vi "scan time(SubVI).vi"(0 "total time":dbl=10.0, 5 "config":T1={"initialize"=enum."SR830", "6221"={"6221 Resource"="GPIB0::24::INSTR", "Delta status"=FALSE, "电流|RMS(A)"=0.0}, "SR830+6221"={"source"=0, "Current(A)"=0.0, "阻抗(Ohm)"=0.0, "SR830 1"=FALSE, "SR830 2"=FALSE, "SR830 3"=FALSE, "SR830 4"=FALSE, "VISA 1"="", "VISA 2"="", "VISA 3"="", "VISA 4"="", "Reserve 1"=0, "Reserve 2"=-1, "Reserve 3"=-1, "Reserve 4"=-1, "Sensitivity 1"=-1, "Sensitivity 2"=0, "Sensitivity 3"=-1, "Sensitivity 4"=-1, "量程入 1"=0, "量程入 2"=0, "量程入 3"=0, "量程入 4"=0}, "2400"={"2400"=FALSE, "VISA"="", "Output Level (0)"=1e-05, "Compliance  Level (0.1)"=10.0, "ch"=[]}, "ch"={"ch"=[], "current"=[], "change?"=[], "holding current\nwhen change ch?"=FALSE}, "Instrument"={"325 Resource "="GPIB0::13::INSTR", "Input (0:A) 325"=0, "Heater Output (1:1) 325"=1, "340 Resource"="GPIB0::14::INSTR", "Input (0:A) 340"=0, "Loop (0: 1)"=0, "Input (0:B) 340"=1, "Loop (1: 1)"=0, "340 Status"=refnum, "Instrument Type"=enum."PPMS-Rotate", "quantum design"=refnum, "semaphore 325"=refnum, "TCP master instance"=refnum, "M24C Resource"="GPIB0::24::INSTR", "4G supply"="GPIB0::24::INSTR", "Temp Status 24C"=refnum, "Temp"=refnum, "9T信号"=refnum, "limit"={"Field limit"=0.0, "Field rate limit"=0.0, "Temp limit"=0.0, "Temp low limit"=0.0, "Temp rate limit "=0.0}, "4g supply status"=refnum, "vi路径"="", "in-plane"="", "out-plane"="", "in-plane signal"=FALSE, "out-plane signal"=FALSE, "in plane 信号"=refnum, "pzt volt"=refnum, "Aborting"=refnum, "数据文件"=refnum, "warning"=refnum, "750 visa"="", "750 rotate"="", "335 Status 2"=refnum, "335 Resource "="GPIB0::24::INSTR", "Input (0:A) 335"=0, "Input (0:B) 335"=1, "Heater Output (1:1) 335"=1, "semaphore 340"=refnum, "semaphore 335"=refnum, "325 Status"=refnum, "semaphore 750"=refnum, "750 field status"=refnum, "camg 振荡状态"=refnum, "列表框"=refnum, "编辑列表框？"=refnum, "camg Rate"=refnum, "行数"=refnum, "TM620"="TCPIP0::192.168.1.5::4266::SOCKET"}, "2614B"={"2614B chA"=FALSE, "2614B chB"=FALSE, "VISA"=""}, "33522b"={"33522b resource name"="", "零电压"=0.0, "最大电压"=148.0, "间隔"=4.0, "最小电压"=-48.0, "loop"=0.0}, "gating type"=enum."2614(daul)", "层数"=0, "行数"=0, "是否处理"=[]} {"Instrument"."Loop (1: 1)" items=["1"=1, "2"=2]; "Instrument"."Loop (0: 1)" items=["1"=1, "2"=2]; "Instrument"."Input (0:B) 340" items=["A", "B", "C", "D"]; "Instrument"."Heater Output (1:1) 335" items=["1"=1, "2"=2]; "Instrument"."Input (0:B) 335" items=["A", "B"]; "Instrument"."Input (0:A) 335" items=["A", "B"]; "Instrument"."Heater Output (1:1) 325" items=["1"=1, "2"=2]; "Instrument"."Input (0:A) 325" items=["A", "B"]; "Instrument"."Input (0:A) 340" items=["1"=1, "2"=2]; "SR830+6221"."Sensitivity 4" items=["Auto Gain"=-1, "2 nV/fA"=0, "5 nV/fA"=1, "10 nV/fA"=2, "20 nV/fA"=3, "50 nV/fA"=4, "100 nV/fA"=5, "200 nV/fA"=6, "500 nV/fA"=7, "1 uV/pA"=8, "2 uV/pA"=9, "5 uV/pA"=10, "10 uV/pA"=11, "20 uV/pA"=12, "50 uV/pA"=13, "100 uV/pA"=14, "200 uV/pA"=15, "500 uV/pA"=16, "1 mV/nA"=17, "2 mV/nA"=18, "5 mV/nA"=19, "10 mV/nA"=20, "20 mV/nA"=21, "50 mV/nA"=22, "100 mV/nA"=23, "200 mV/nA"=24, "500 mV/mA"=25, "1 V/uA"=26]; "SR830+6221"."Sensitivity 3" items=["Auto Gain"=-1, "2 nV/fA"=0, "5 nV/fA"=1, "10 nV/fA"=2, "20 nV/fA"=3, "50 nV/fA"=4, "100 nV/fA"=5, "200 nV/fA"=6, "500 nV/fA"=7, "1 uV/pA"=8, "2 uV/pA"=9, "5 uV/pA"=10, "10 uV/pA"=11, "20 uV/pA"=12, "50 uV/pA"=13, "100 uV/pA"=14, "200 uV/pA"=15, "500 uV/pA"=16, "1 mV/nA"=17, "2 mV/nA"=18, "5 mV/nA"=19, "10 mV/nA"=20, "20 mV/nA"=21, "50 mV/nA"=22, "100 mV/nA"=23, "200 mV/nA"=24, "500 mV/mA"=25, "1 V/uA"=26]; "SR830+6221"."Sensitivity 1" items=["Auto Gain"=-1, "2 nV/fA"=0, "5 nV/fA"=1, "10 nV/fA"=2, "20 nV/fA"=3, "50 nV/fA"=4, "100 nV/fA"=5, "200 nV/fA"=6, "500 nV/fA"=7, "1 uV/pA"=8, "2 uV/pA"=9, "5 uV/pA"=10, "10 uV/pA"=11, "20 uV/pA"=12, "50 uV/pA"=13, "100 uV/pA"=14, "200 uV/pA"=15, "500 uV/pA"=16, "1 mV/nA"=17, "2 mV/nA"=18, "5 mV/nA"=19, "10 mV/nA"=20, "20 mV/nA"=21, "50 mV/nA"=22, "100 mV/nA"=23, "200 mV/nA"=24, "500 mV/mA"=25, "1 V/uA"=26]; "SR830+6221"."Sensitivity 2" items=["Auto Gain"=-1, "2 nV/fA"=0, "5 nV/fA"=1, "10 nV/fA"=2, "20 nV/fA"=3, "50 nV/fA"=4, "100 nV/fA"=5, "200 nV/fA"=6, "500 nV/fA"=7, "1 uV/pA"=8, "2 uV/pA"=9, "5 uV/pA"=10, "10 uV/pA"=11, "20 uV/pA"=12, "50 uV/pA"=13, "100 uV/pA"=14, "200 uV/pA"=15, "500 uV/pA"=16, "1 mV/nA"=17, "2 mV/nA"=18, "5 mV/nA"=19, "10 mV/nA"=20, "20 mV/nA"=21, "50 mV/nA"=22, "100 mV/nA"=23, "200 mV/nA"=24, "500 mV/mA"=25, "1 V/uA"=26]; "SR830+6221"."Reserve 4" items=["Auto Gain"=-1, "2 nV/fA"=0, "5 nV/fA"=1, "10 nV/fA"=2, "20 nV/fA"=3, "50 nV/fA"=4, "100 nV/fA"=5, "200 nV/fA"=6, "500 nV/fA"=7, "1 uV/pA"=8, "2 uV/pA"=9, "5 uV/pA"=10, "10 uV/pA"=11, "20 uV/pA"=12, "50 uV/pA"=13, "100 uV/pA"=14, "200 uV/pA"=15, "500 uV/pA"=16, "1 mV/nA"=17, "2 mV/nA"=18, "5 mV/nA"=19, "10 mV/nA"=20, "20 mV/nA"=21, "50 mV/nA"=22, "100 mV/nA"=23, "200 mV/nA"=24, "500 mV/mA"=25, "1 V/uA"=26]; "SR830+6221"."Reserve 3" items=["Auto Reserve"=-1, "High Reserve"=0, "Normal"=1, "Low Noise"=2]; "SR830+6221"."Reserve 2" items=["Auto Reserve"=-1, "High Reserve"=0, "Normal"=1, "Low Noise"=2]; "SR830+6221"."Reserve 1" items=["Auto Reserve"=-1, "High Reserve"=0, "Normal"=1, "Low Noise"=2]; "SR830+6221"."source" items=["SR830 1", "SR830 2", "SR830 3", "SR830 4"]}, 9 "steps number":i32, 12 "data":refnum<queue>) -> (4 "输出簇":T1={"initialize"=enum."SR830", "6221"={"6221 Resource"="GPIB0::24::INSTR", "Delta status"=FALSE, "电流|RMS(A)"=0.0}, "SR830+6221"={"source"=0, "Current(A)"=0.0, "阻抗(Ohm)"=0.0, "SR830 1"=FALSE, "SR830 2"=FALSE, "SR830 3"=FALSE, "SR830 4"=FALSE, "VISA 1"="", "VISA 2"="", "VISA 3"="", "VISA 4"="", "Reserve 1"=0, "Reserve 2"=-1, "Reserve 3"=-1, "Reserve 4"=-1, "Sensitivity 1"=-1, "Sensitivity 2"=0, "Sensitivity 3"=-1, "Sensitivity 4"=-1, "量程入 1"=0, "量程入 2"=0, "量程入 3"=0, "量程入 4"=0}, "2400"={"2400"=FALSE, "VISA"="", "Output Level (0)"=1e-05, "Compliance  Level (0.1)"=10.0, "ch"=[]}, "ch"={"ch"=[], "current"=[], "change?"=[], "holding current\nwhen change ch?"=FALSE}, "Instrument"={"325 Resource "="GPIB0::13::INSTR", "Input (0:A) 325"=0, "Heater Output (1:1) 325"=1, "340 Resource"="GPIB0::14::INSTR", "Input (0:A) 340"=0, "Loop (0: 1)"=0, "Input (0:B) 340"=1, "Loop (1: 1)"=0, "340 Status"=refnum, "Instrument Type"=enum."PPMS-Rotate", "quantum design"=refnum, "semaphore 325"=refnum, "TCP master instance"=refnum, "M24C Resource"="GPIB0::24::INSTR", "4G supply"="GPIB0::24::INSTR", "Temp Status 24C"=refnum, "Temp"=refnum, "9T信号"=refnum, "limit"={"Field limit"=0.0, "Field rate limit"=0.0, "Temp limit"=0.0, "Temp low limit"=0.0, "Temp rate limit "=0.0}, "4g supply status"=refnum, "vi路径"="", "in-plane"="", "out-plane"="", "in-plane signal"=FALSE, "out-plane signal"=FALSE, "in plane 信号"=refnum, "pzt volt"=refnum, "Aborting"=refnum, "数据文件"=refnum, "warning"=refnum, "750 visa"="", "750 rotate"="", "335 Status 2"=refnum, "335 Resource "="GPIB0::24::INSTR", "Input (0:A) 335"=0, "Input (0:B) 335"=1, "Heater Output (1:1) 335"=1, "semaphore 340"=refnum, "semaphore 335"=refnum, "325 Status"=refnum, "semaphore 750"=refnum, "750 field status"=refnum, "camg 振荡状态"=refnum, "列表框"=refnum, "编辑列表框？"=refnum, "camg Rate"=refnum, "行数"=refnum, "TM620"="TCPIP0::192.168.1.5::4266::SOCKET"}, "2614B"={"2614B chA"=FALSE, "2614B chB"=FALSE, "VISA"=""}, "33522b"={"33522b resource name"="", "零电压"=0.0, "最大电压"=148.0, "间隔"=4.0, "最小电压"=-48.0, "loop"=0.0}, "gating type"=enum."2614(daul)", "层数"=0, "行数"=0, "是否处理"=[]} {"Instrument"."Loop (1: 1)" items=["1"=1, "2"=2]; "Instrument"."Loop (0: 1)" items=["1"=1, "2"=2]; "Instrument"."Input (0:B) 340" items=["A", "B", "C", "D"]; "Instrument"."Heater Output (1:1) 335" items=["1"=1, "2"=2]; "Instrument"."Input (0:B) 335" items=["A", "B"]; "Instrument"."Input (0:A) 335" items=["A", "B"]; "Instrument"."Heater Output (1:1) 325" items=["1"=1, "2"=2]; "Instrument"."Input (0:A) 325" items=["A", "B"]; "Instrument"."Input (0:A) 340" items=["1"=1, "2"=2]; "SR830+6221"."Sensitivity 4" items=["Auto Gain"=-1, "2 nV/fA"=0, "5 nV/fA"=1, "10 nV/fA"=2, "20 nV/fA"=3, "50 nV/fA"=4, "100 nV/fA"=5, "200 nV/fA"=6, "500 nV/fA"=7, "1 uV/pA"=8, "2 uV/pA"=9, "5 uV/pA"=10, "10 uV/pA"=11, "20 uV/pA"=12, "50 uV/pA"=13, "100 uV/pA"=14, "200 uV/pA"=15, "500 uV/pA"=16, "1 mV/nA"=17, "2 mV/nA"=18, "5 mV/nA"=19, "10 mV/nA"=20, "20 mV/nA"=21, "50 mV/nA"=22, "100 mV/nA"=23, "200 mV/nA"=24, "500 mV/mA"=25, "1 V/uA"=26]; "SR830+6221"."Sensitivity 3" items=["Auto Gain"=-1, "2 nV/fA"=0, "5 nV/fA"=1, "10 nV/fA"=2, "20 nV/fA"=3, "50 nV/fA"=4, "100 nV/fA"=5, "200 nV/fA"=6, "500 nV/fA"=7, "1 uV/pA"=8, "2 uV/pA"=9, "5 uV/pA"=10, "10 uV/pA"=11, "20 uV/pA"=12, "50 uV/pA"=13, "100 uV/pA"=14, "200 uV/pA"=15, "500 uV/pA"=16, "1 mV/nA"=17, "2 mV/nA"=18, "5 mV/nA"=19, "10 mV/nA"=20, "20 mV/nA"=21, "50 mV/nA"=22, "100 mV/nA"=23, "200 mV/nA"=24, "500 mV/mA"=25, "1 V/uA"=26]; "SR830+6221"."Sensitivity 1" items=["Auto Gain"=-1, "2 nV/fA"=0, "5 nV/fA"=1, "10 nV/fA"=2, "20 nV/fA"=3, "50 nV/fA"=4, "100 nV/fA"=5, "200 nV/fA"=6, "500 nV/fA"=7, "1 uV/pA"=8, "2 uV/pA"=9, "5 uV/pA"=10, "10 uV/pA"=11, "20 uV/pA"=12, "50 uV/pA"=13, "100 uV/pA"=14, "200 uV/pA"=15, "500 uV/pA"=16, "1 mV/nA"=17, "2 mV/nA"=18, "5 mV/nA"=19, "10 mV/nA"=20, "20 mV/nA"=21, "50 mV/nA"=22, "100 mV/nA"=23, "200 mV/nA"=24, "500 mV/mA"=25, "1 V/uA"=26]; "SR830+6221"."Sensitivity 2" items=["Auto Gain"=-1, "2 nV/fA"=0, "5 nV/fA"=1, "10 nV/fA"=2, "20 nV/fA"=3, "50 nV/fA"=4, "100 nV/fA"=5, "200 nV/fA"=6, "500 nV/fA"=7, "1 uV/pA"=8, "2 uV/pA"=9, "5 uV/pA"=10, "10 uV/pA"=11, "20 uV/pA"=12, "50 uV/pA"=13, "100 uV/pA"=14, "200 uV/pA"=15, "500 uV/pA"=16, "1 mV/nA"=17, "2 mV/nA"=18, "5 mV/nA"=19, "10 mV/nA"=20, "20 mV/nA"=21, "50 mV/nA"=22, "100 mV/nA"=23, "200 mV/nA"=24, "500 mV/mA"=25, "1 V/uA"=26]; "SR830+6221"."Reserve 4" items=["Auto Gain"=-1, "2 nV/fA"=0, "5 nV/fA"=1, "10 nV/fA"=2, "20 nV/fA"=3, "50 nV/fA"=4, "100 nV/fA"=5, "200 nV/fA"=6, "500 nV/fA"=7, "1 uV/pA"=8, "2 uV/pA"=9, "5 uV/pA"=10, "10 uV/pA"=11, "20 uV/pA"=12, "50 uV/pA"=13, "100 uV/pA"=14, "200 uV/pA"=15, "500 uV/pA"=16, "1 mV/nA"=17, "2 mV/nA"=18, "5 mV/nA"=19, "10 mV/nA"=20, "20 mV/nA"=21, "50 mV/nA"=22, "100 mV/nA"=23, "200 mV/nA"=24, "500 mV/mA"=25, "1 V/uA"=26]; "SR830+6221"."Reserve 3" items=["Auto Reserve"=-1, "High Reserve"=0, "Normal"=1, "Low Noise"=2]; "SR830+6221"."Reserve 2" items=["Auto Reserve"=-1, "High Reserve"=0, "Normal"=1, "Low Noise"=2]; "SR830+6221"."Reserve 1" items=["Auto Reserve"=-1, "High Reserve"=0, "Normal"=1, "Low Noise"=2]; "SR830+6221"."source" items=["SR830 1", "SR830 2", "SR830 3", "SR830 4"]}, 6 "错误输出":errorcluster)   [LabVIEW 2019, in "Scan.lvlib"]
uses:
  Scan.lvlib
  ctl/config.ctl
  <vilib>/NI/Modbus Library/API/Master/Modbus Master.lvclass
  ctl/initialize.ctl
  ctl/Instrument.ctl
  ctl/335 state.ctl
  ctl/Instrument Type.ctl
  C:/Users/fuyang/Desktop/postdoctor/labview/labview-measure/lib/QDInstrument.dll
  lib/QDInstrument.dll
  ctl/limit.ctl
  ctl/9T mag field stauts.ctl
  ctl/warning.ctl
  ctl/Gating type.ctl
  User lib.lvlib
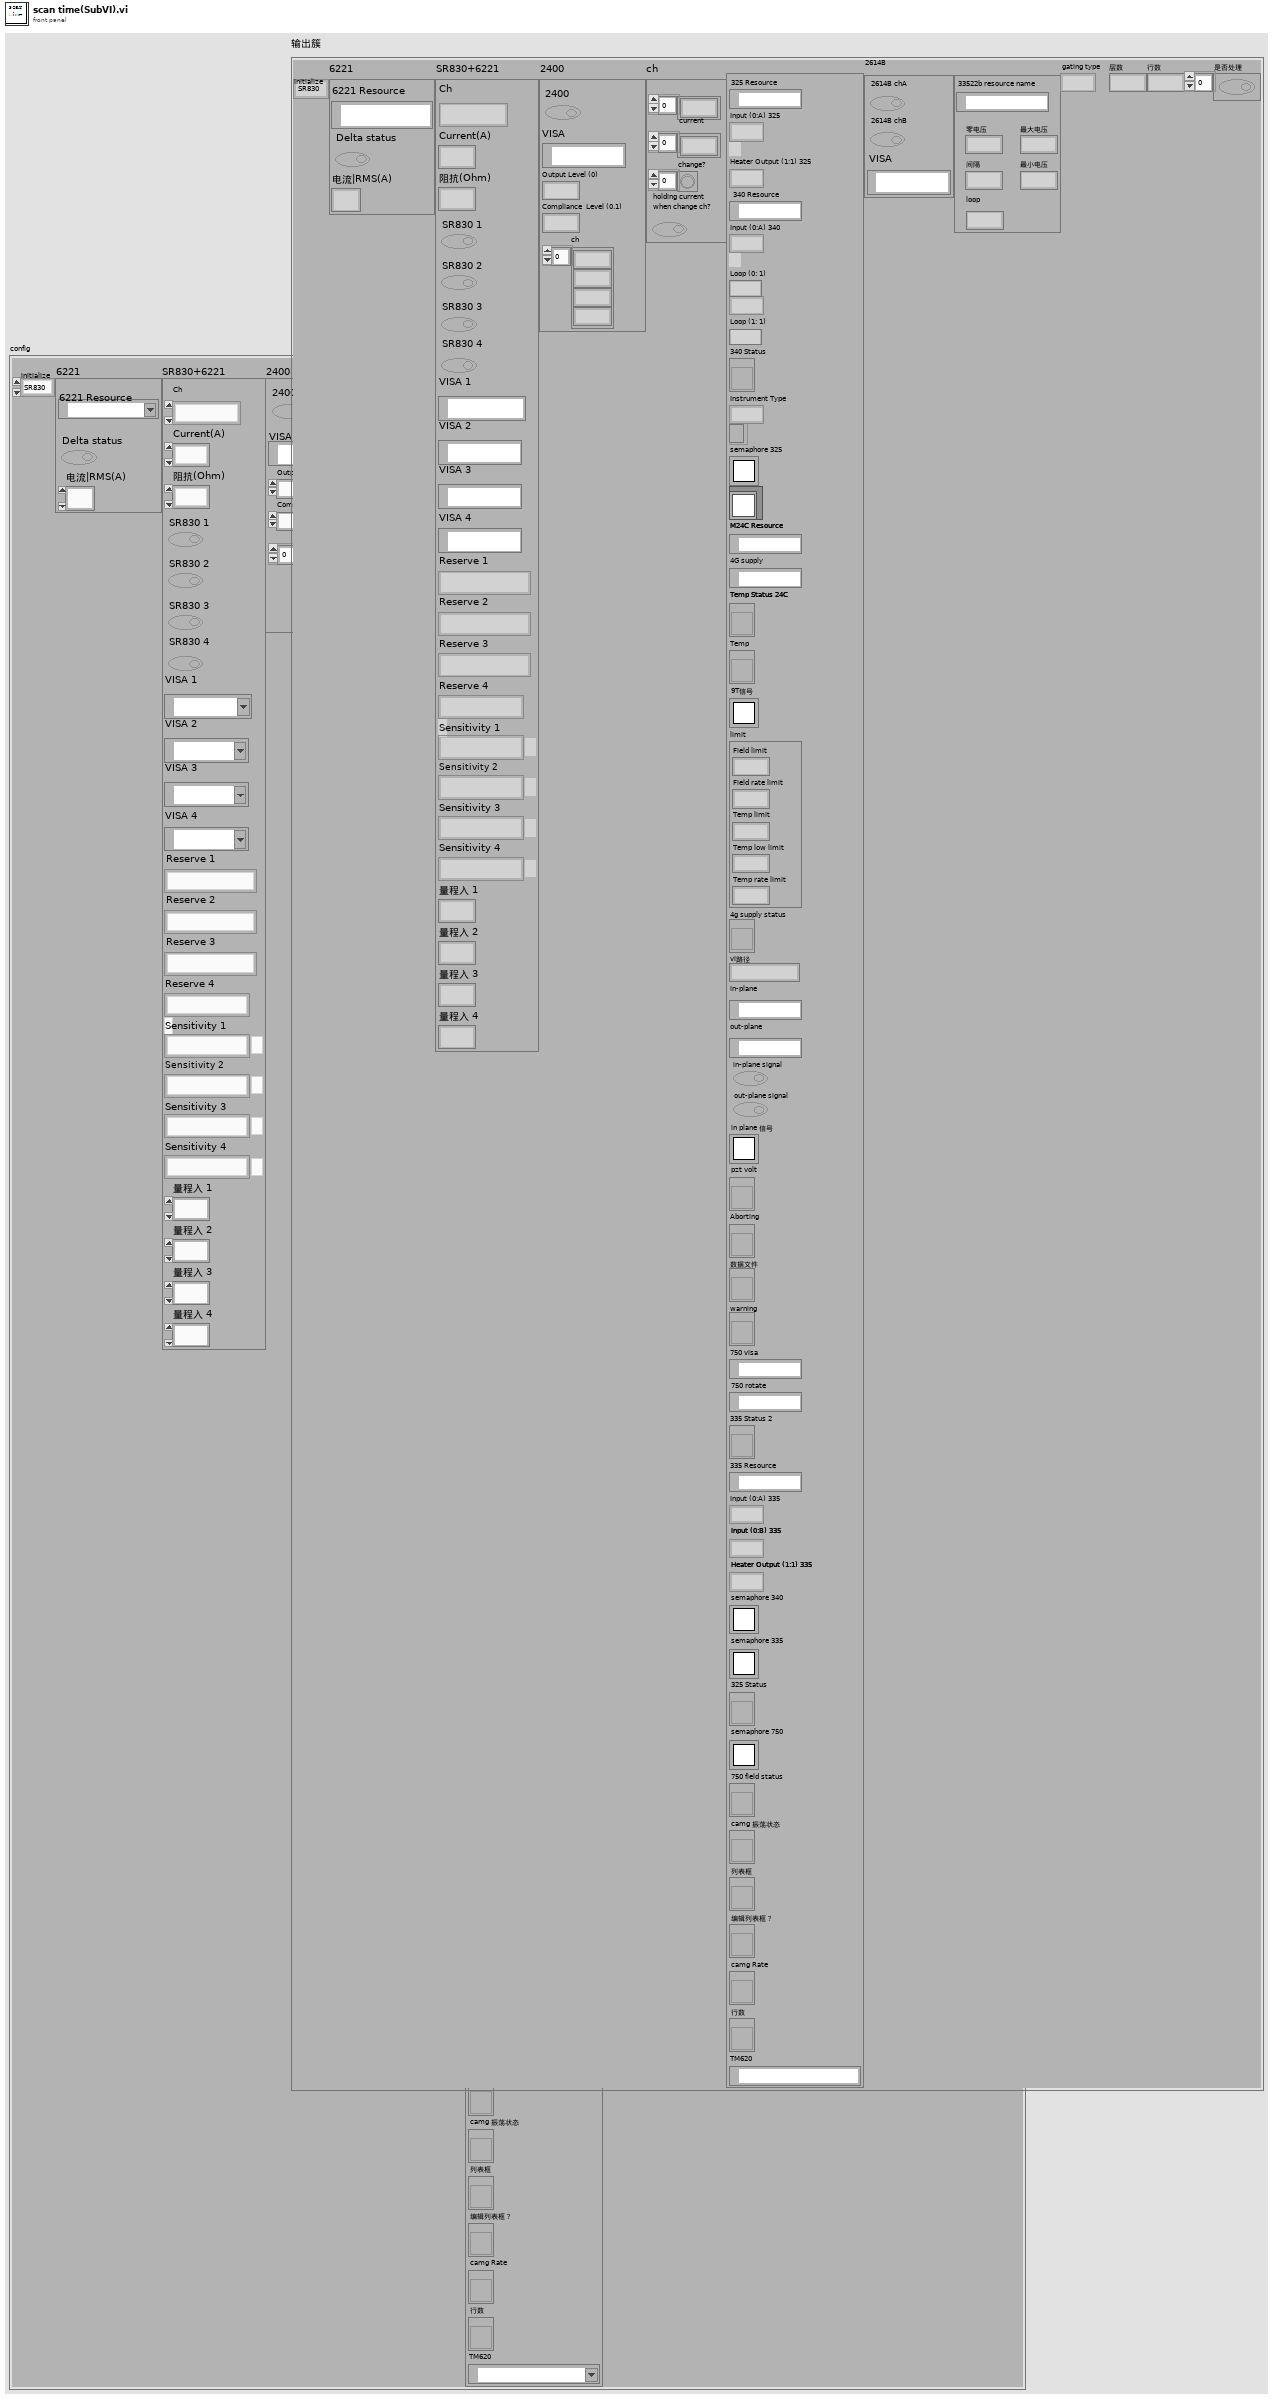
[diagram p1: front panel]
types:
  T1 = typedef "config.ctl" = cluster{"initialize":T2, "6221":cluster{"6221 Resource":refnum<visa-resource-name>, "Delta status":bool, "电流|RMS(A)":dbl}, "SR830+6221":cluster{"source":u16, "Current(A)":dbl, "阻抗(Ohm)":dbl, "SR830 1":bool, "SR830 2":bool, "SR830 3":bool, "SR830 4":bool, "VISA 1":refnum<visa-resource-name>, "VISA 2":refnum<visa-resource-name>, "VISA 3":refnum<visa-resource-name>, "VISA 4":refnum<visa-resource-name>, "Reserve 1":i16, "Reserve 2":i16, "Reserve 3":i16, "Reserve 4":i16, "Sensitivity 1":i16, "Sensitivity 2":i16, "Sensitivity 3":i16, "Sensitivity 4":i16, "量程入 1":i32, "量程入 2":i32, "量程入 3":i32, "量程入 4":i32}, "2400":cluster{"2400":bool, "VISA":refnum<visa-resource-name>, "Output Level (0)":dbl, "Compliance  Level (0.1)":dbl, "ch":i32[]}, "ch":cluster{"ch":i32[], "current":dbl[], "change?":bool[], "holding current\nwhen change ch?":bool}, "Instrument":T3, "2614B":cluster{"2614B chA":bool, "2614B chB":bool, "VISA":refnum<visa-resource-name>}, "33522b":cluster{"33522b resource name":refnum<visa-resource-name>, "零电压":dbl, "最大电压":dbl, "间隔":dbl, "最小电压":dbl, "loop":dbl}, "gating type":T7, "层数":i32, "行数":i32, "是否处理":bool[]}
  T2 = typedef "initialize.ctl" = enum16{"SR830", "keithley6221-SR830", "Delta", "Delta-tunnelling", "keithley6221-2182-DC", "PZT", "4200"}
  T3 = typedef "Instrument.ctl" = cluster{"325 Resource ":refnum<visa-resource-name>, "Input (0:A) 325":u16, "Heater Output (1:1) 325":u16, "340 Resource":refnum<visa-resource-name>, "Input (0:A) 340":u16, "Loop (0: 1)":u16, "Input (0:B) 340":u16, "Loop (1: 1)":u16, "340 Status":refnum<vi>, "Instrument Type":T4, "quantum design":refnum<k24>, "semaphore 325":T5, "TCP master instance":refnum<class "Modbus Master.lvclass">, "M24C Resource":refnum<visa-resource-name>, "4G supply":refnum<visa-resource-name>, "Temp Status 24C":refnum<vi>, "Temp":refnum<vi>, "9T信号":T5, "limit":T6, "4g supply status":refnum<vi>, "vi路径":string, "in-plane":refnum<visa-resource-name>, "out-plane":refnum<visa-resource-name>, "in-plane signal":bool, "out-plane signal":bool, "in plane 信号":T5, "pzt volt":refnum<vi>, "Aborting":refnum<vi>, "数据文件":refnum<vi>, "warning":refnum<vi>, "750 visa":refnum<visa-resource-name>, "750 rotate":refnum<visa-resource-name>, "335 Status 2":refnum<vi>, "335 Resource ":refnum<visa-resource-name>, "Input (0:A) 335":u16, "Input (0:B) 335":u16, "Heater Output (1:1) 335":u16, "semaphore 340":T5, "semaphore 335":T5, "325 Status":refnum<vi>, "semaphore 750":T5, "750 field status":refnum<vi>, "camg 振荡状态":refnum<vi>, "列表框":refnum<vi>, "编辑列表框？":refnum<vi>, "camg Rate":refnum<vi>, "行数":refnum<vi>, "TM620":refnum<visa-resource-name>}
  T4 = typedef "Instrument Type.ctl" = enum16{"PPMS", "VersaLab", "DynaCool", "SVSM", "PPMS-Rotate", "Lakeshore335", "lengtou2", "9T mag old", "9T cmag", "9T cmag DAC", "9T cmag rotate", "test"}
  T5 = typedef "Semaphore RefNum" = refnum<k1>
  T6 = typedef "limit.ctl" = cluster{"Field limit":dbl, "Field rate limit":dbl, "Temp limit":dbl, "Temp low limit":dbl, "Temp rate limit ":dbl}
  T7 = typedef "Gating type.ctl" = enum32{"null", "2614(daul)", "2400", "6517B"}
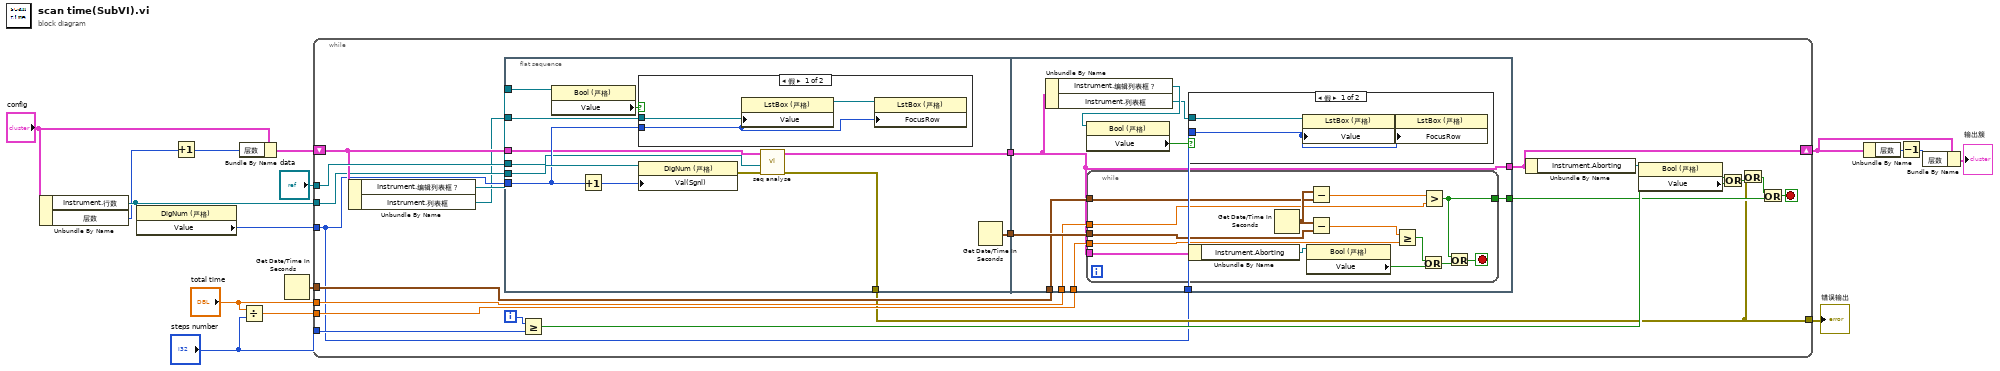
[diagram p0: block diagram]
diagram:
  n1 = Unbundle By Name("config") -> ("Instrument.行数"=w9:refnum<vi>, "层数"=w8:i32)
  n2 = property class="DigNum (严格)"(reference=w9) -> ("Value"=w10:i32)  [unwired: 1 in, 2 out]
  n3 = Increment(x=w8) -> (x+1=w6:i32)
  n4 = Bundle By Name(cluster="config", "层数"=w6) -> (w5:T1)
  n5 = Divide(x="total time", y="steps number") -> (x/y=w15:dbl)
  n6 = Get Date/Time In Seconds() -> (seconds since 1Jan1904=w12:timestamp)
  n7 = while {
    tunnel: "steps number" -> [w36]
    tunnel: "data" -> [w38]
    tunnel: w15 -> [w31]
    tunnel: [w20] -> w14
    tunnel: w12 -> [w32]
    tunnel: "total time" -> [w27]
    shift-right: [w24] -> w2
    shift-left: w5 -> [w22]
    tunnel: w10 -> [w18]
    tunnel: w9 -> [w21]
    i -> [w35]
    stop <- w28 stop-if-true
    n8 = Unbundle By Name(w22) -> ("Instrument.编辑列表框？"=w19:refnum<vi>, "Instrument.列表框"=w17:refnum<vi>)
    n9 = flat-sequence {
      tunnel: w38 -> [w39]
      tunnel: w22 -> [w42]
      tunnel: [w50] -> w33
      tunnel: [w41] -> w23
      tunnel: w21 -> [w46]
      tunnel: w19 -> [w45]
      tunnel: w17 -> [w44]
      tunnel: w18 -> [w43]
      tunnel: [w40] -> w20
      tunnel: [w54] -> w24
      tunnel: w31 -> [w62]
      tunnel: w33 -> [w63]
      tunnel: w32 -> [w61]
      tunnel: w27 -> [w60]
      tunnel: [w59] -> w29
      tunnel: w23 -> [w54]
      tunnel: w18 -> [w57]
      frame #0 {
        n10 = property class="Bool (严格)"(reference=w45) -> ("Value"=w47:bool)  [unwired: 1 in, 2 out]
        n11 = Increment(x=w43) -> (x+1=w49:i32)
        n12 = case shown="假" w47 {
          tunnel: w43 -> [w53 _]
          tunnel: w44 -> [w51 _]
          frame False {
            n13 = property on="属性节点" class="LstBox (严格)"(reference=w51, "Value"=w53) -> (reference out=w52:refnum<vi>)  [unwired: 1 in, 1 out]
            n14 = property on="属性节点" class="LstBox (严格)"(reference=w52, "FocusRow"=w53) -> ()  [unwired: 1 in, 2 out]
          }
          frame True {
          }
        }
        n15 = property class="DigNum (严格)"(reference=w46, "Val(Sgnl)"=w49) -> (error out=w48:errorcluster)  [unwired: 1 in, 1 out]
        n16 = call "seq analyse.vi"("config"=w42, "数据队列"=w39, "错误输入"=w48) -> ("config out"=w41:T1, "错误输出"=w40:errorcluster)  [unwired: 6 in]
        n17 = Get Date/Time In Seconds() -> (seconds since 1Jan1904=w50:timestamp)
      }
      frame #1 {
        n18 = Unbundle By Name(w54) -> ("Instrument.编辑列表框？"=w56:refnum<vi>, "Instrument.列表框"=w55:refnum<vi>)
        n19 = property class="Bool (严格)"(reference=w56) -> ("Value"=w58:bool)  [unwired: 1 in, 2 out]
        n20 = while {
          tunnel: w63 -> [w77]
          tunnel: w62 -> [w79]
          tunnel: w54 -> [w69]
          tunnel: w61 -> [w75]
          tunnel: w60 -> [w73]
          tunnel: [w72] -> w59
          stop <- w70 stop-if-true
          n21 = Unbundle By Name(w69) -> ("Instrument.Aborting"=w68:refnum<vi>)
          n22 = Get Date/Time In Seconds() -> (seconds since 1Jan1904=w76:timestamp)
          n23 = property class="Bool (严格)"(reference=w68) -> ("Value"=w67:bool)  [unwired: 1 in, 2 out]
          n24 = Subtract(x=w76, y=w75) -> (x-y=w74:dbl)
          n25 = Subtract(x=w76, y=w77) -> (x-y=w80:dbl)
          n26 = Greater Or Equal?(x=w80, y=w79) -> (x >= y?=w78:bool)
          n27 = Or(x=w78, y=w67) -> (x .or. y?=w71:bool)
          n28 = Greater?(x=w74, y=w73) -> (0:w72:bool)
          n29 = Or(x=w72, y=w71) -> (x .or. y?=w70:bool)
        }
        n30 = case shown="假" w58 {
          tunnel: w57 -> [w66 _]
          tunnel: w55 -> [w64 _]
          frame False {
            n31 = property on="属性节点" class="LstBox (严格)"(reference=w64, "Value"=w66) -> (reference out=w65:refnum<vi>)  [unwired: 1 in, 1 out]
            n32 = property on="属性节点" class="LstBox (严格)"(reference=w65, "FocusRow"=w66) -> ()  [unwired: 1 in, 2 out]
          }
          frame True {
          }
        }
      }
    }
    n33 = Greater Or Equal?(x=w35, y=w36) -> (x >= y?=w37:bool)
    n34 = Unbundle By Name(w24) -> ("Instrument.Aborting"=w26:refnum<vi>)
    n35 = property class="Bool (严格)"(reference=w26) -> ("Value"=w25:bool)  [unwired: 1 in, 2 out]
    n36 = Or(x=w37, y=w25) -> (x .or. y?=w34:bool)
    n37 = Or(x=w20, y=w34) -> (x .or. y?=w30:bool)
    n38 = Or(x=w30, y=w29) -> (x .or. y?=w28:bool)
  }
  "错误输出" <- w14
  n39 = Unbundle By Name(w2) -> ("层数"=w4:i32)
  n40 = Decrement(x=w4) -> (x-1=w3:i32)
  n41 = Bundle By Name(cluster=w2, "层数"=w3) -> (→"输出簇":T1)
